vi "Test Pass if Expected Call Made.vi"(8 "error in (no error)":errorcluster, 11 "Test Case In":refnum<class "One or More Expectation Test.lvclass">) -> (0 "error out":errorcluster, 3 "Test Case Out":refnum<class "One or More Expectation Test.lvclass">)   [LabVIEW 2020, in "One or More Expectation Test.lvclass"]
uses:
  One or More Expectation Test.lvclass
  C:/Program Files (x86)/National Instruments/LabVIEW 2020/vi.lib/Astemes/LUnit/Test Case.lvclass
  Test Interface Mock/Test Interface Mock.lvclass
  C:/git/astemes-lmock/sandbox/Mock/Mock.lvclass
  One or More Expectation Test.lvclass/One or More Expectation Test.ctl
  Expectation Test/Expectation Test.lvclass
  C:/git/astemes-lmock/sandbox/Test Interface Mock/Test Interface Mock.lvclass
  C:/git/astemes-lmock/sandbox/Test Interface/Test Interface.lvclass
  One or More of/One Of/One or More.lvclass
  C:/git/astemes-lmock/sandbox/Expectation Test/Expectation Test.lvclass
  C:/Program Files (x86)/National Instruments/LabVIEW 2020/vi.lib/Astemes/LUnit/LUnit Runnable.lvclass
  C:/git/astemes-lmock/sandbox/One or More Test/One or More Expectation Test.lvclass
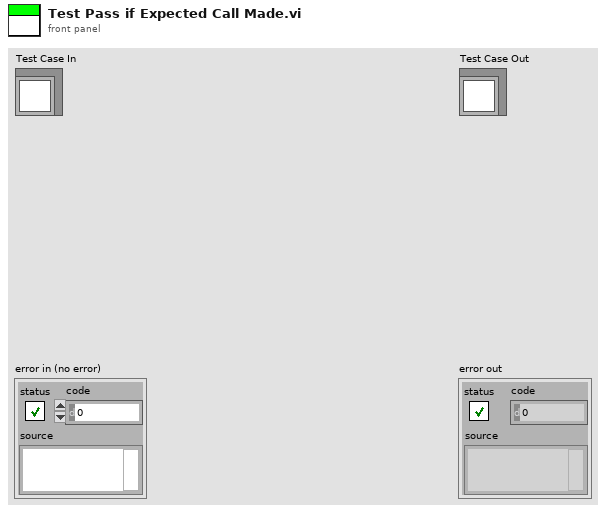
[diagram p1: front panel]
types:
  T1 = enum16{"", "Passed", "Failed", "Error", "Skipped", "Setup Error", "Broken", "Teardown Error"}
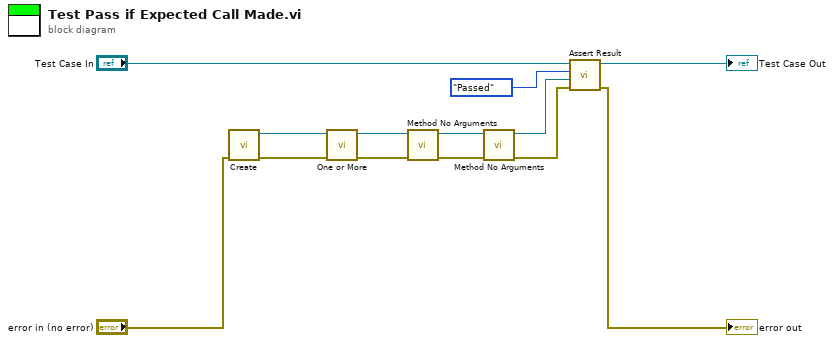
[diagram p0: block diagram]
diagram:
  n1 = call "Create.vi"("error in (no error)"="error in (no error)") -> ("error out"=w9:errorcluster, "Test Interface Mock Out"=w7:refnum<class "Test Interface Mock.lvclass">)  [unwired: 9 in]
  n2 = call "One or More.vi"("error in (no error)"=w9, "Mock in"=w7) -> ("error out"=w8:errorcluster, "Mock out"=w6:refnum<class "Test Interface Mock.lvclass">)  [unwired: 8 in]
  n3 = call-dynamic "Method No Arguments.vi"("error in (no error)"=w8, "Mock In"=w6) -> ("error out"=w5:errorcluster, "Mock Out"=w2:refnum<class "Test Interface Mock.lvclass">)  [unwired: 8 in]
  n4 = call-dynamic "Method No Arguments.vi"("error in (no error)"=w5, "Mock In"=w2) -> ("error out"=w3:errorcluster, "Mock Out"=w1:refnum<class "Test Interface Mock.lvclass">)  [unwired: 8 in]
  n5 = call "Assert Result.vi"("error in (no error)"=w3, "Mock"=w1, "Status"=T1."Passed", "LUnit Test Case In"="Test Case In") -> ("error out"=→"error out":errorcluster, "LUnit Test Case In"=→"Test Case Out":refnum<class "One or More Expectation Test.lvclass">)  [unwired: 6 in]
